vi "Read_Data.vi"(2 "item":string, 3 "topic":string="VAR_TABLE", 4 "service":string="ROBCOMM") -> (0 "Error?":bool, 1 "data":string)   [LabVIEW 2012]
panel:
  # "If read var throws an error. Check to make sure the variable exists in robot arm memory \nand if not create."
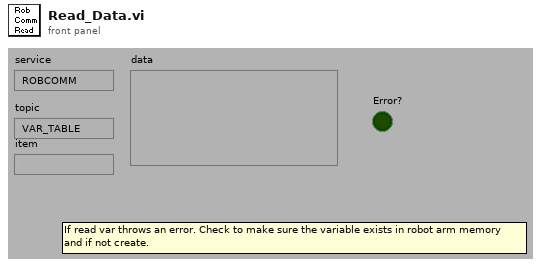
[diagram p1: front panel]
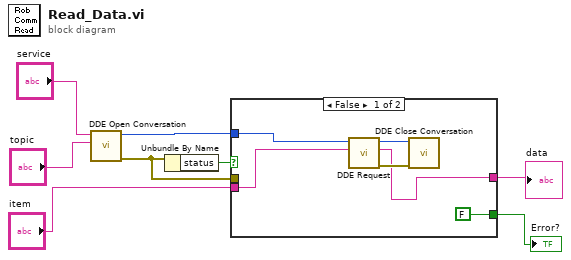
[diagram p0: block diagram]
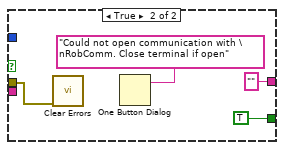
[diagram p2: hidden frame]
diagram:
  n1 = call <vilib>:"DDE Open Conversation.vi"("topic"="topic", "service"="service") -> ("error out"=w3:errorcluster, "conversation refnum"=w5:u32)  [unwired: 6 in]
  n2 = Unbundle By Name(w3) -> ("status"=w6:bool)
  n3 = case shown="False" w6 {
    tunnel: w5 -> [w14 _]
    tunnel: "item" -> [w13 _]
    tunnel: w3 -> [_ w16]
    tunnel: [w10 "" ("data")] -> w2
    tunnel: [FALSE TRUE] -> w1
    frame False {
      n4 = call <vilib>:"DDE Request.vi"("item"=w13, "conversation refnum in"=w14) -> ("error out"=w12:errorcluster, "data"=w10:string, "conversation refnum out"=w11:u32)  [unwired: 5 in]
      n5 = call <vilib>:"DDE Close Conversation.vi"("error in (no error)"=w12, "conversation refnum"=w11) -> ()  [unwired: 7 in, 1 out]
    }
    frame True {
      n6 = call <vilib>:"Clear Errors.vi"("error in (no error)"=w16) -> ()  [unwired: 6 in, 1 out]
      n7 = One Button Dialog(message="Could not open communication with \nRobComm. Close terminal if open") -> ()  [unwired: 1 in, 1 out]
    }
  }
  "data" <- w2
  "Error?" <- w1
